vi "Agilent PNA Measure2.vi"(0 "VISA session":refnum<visa-resource-name>="GPIB0::16::INSTR", 11 "Error In (no error)":errorcluster) -> (4 "dup VISA session":refnum<visa-resource-name>="GPIB0::16::INSTR", 10 "Sweep Time":dbl=0.19447074 format="%.2p", 15 "Error Out":errorcluster)   [LabVIEW 2018]
doc: "This VI configures the sweep parameters and reads data from the analyzer.\n\nNote: To see the data on the analyzer after running the program, from the front panel click: Trace - Math/Memory - Memory Trace"
uses:
  Agilent PNA Series/Agilent PNA Series.lvlib
panel:
  # "(c) 2005-2015 National Instruments.  ALL RIGHTS RESERVED."
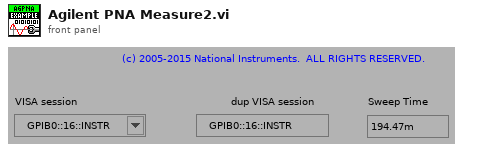
[diagram p1: front panel]
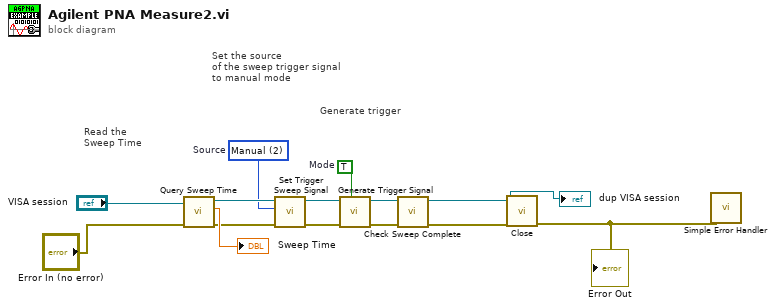
[diagram p0: block diagram]
diagram:
  w6 = TRUE  # Mode
  w7 = u16 2 items=["Immediate", "External", "Manual"]  # Source
  # "Generate trigger"
  # "Read the \nSweep Time"
  # "Set the source \nof the sweep trigger signal \nto manual mode"
  n1 = call "Query Sweep Time.vi"("Error In (no error)"="Error In (no error)", "VISA Resource Name"="VISA session") -> ("Error Out"=w8:errorcluster, "Sweep Time"=→"Sweep Time":dbl, "VISA Resource Name Out"=w9:refnum<visa-resource-name>)  [unwired: 7 in]
  n2 = call "Set Trigger Sweep Signal.vi"("Error In (no error)"=w8, "Source (0: Immediate)"=w7, "VISA session"=w9) -> ("Error Out"=w14:errorcluster, "dup VISA session"=w13:refnum<visa-resource-name>)  [unwired: 7 in]
  n3 = call "Generate Trigger Signal.vi"("Mode (T: Initiate)"=w6, "Error In (no error)"=w14, "VISA Resource Name"=w13) -> ("Error Out"=w10:errorcluster, "VISA Resource Name Out"=w11:refnum<visa-resource-name>)  [unwired: 7 in]
  n4 = call "Check Sweep Complete.vi"("Error In (no error)"=w10, "VISA Resource Name"=w11) -> ("Error Out"=w1:errorcluster, "VISA Resource Name Out"=w2:refnum<visa-resource-name>)  [unwired: 7 in, 1 out]
  "dup VISA session" <- w2
  n5 = call "Close.vi"("Error In (no error)"=w1, "VISA Resource Name"=w2) -> ("Error Out"=w5:errorcluster)  [unwired: 9 in]
  "Error Out" <- w5
  n6 = call <vilib>:"Simple Error Handler.vi"("error in (no error)"=w5) -> ()  [unwired: 4 in, 5 out]
